vi "Set Adv Mov wrapper.vi"(8 "error in (no error)":errorcluster caption="错误输入（无错误）", 9 "pAdvMovObj":T1, 10 "dwCanNodeId":u32, 11 "dwDevIndex":u32) -> (0 "error out":errorcluster caption="错误输出", 1 "pAdvMovObj out":T1, 3 "function return":u32)   [LabVIEW 2016, in "UISimCanFunc_wrapper.lvlib"]
doc: "_declspec (dllexport) DWORD SetAdvMov_wrapper(DWORD dwDevIndex, DWORD dwCanNodeId, P_ADV_MOVE_PARA_OBJ pAdvMovObj);"
uses:
  <userlib>/UISimCanFunc_wrapper/UISimCanFunc_wrapper.lvlib
  <userlib>/UISimCanFunc_wrapper/UISimCanFunc_wrapper.dll
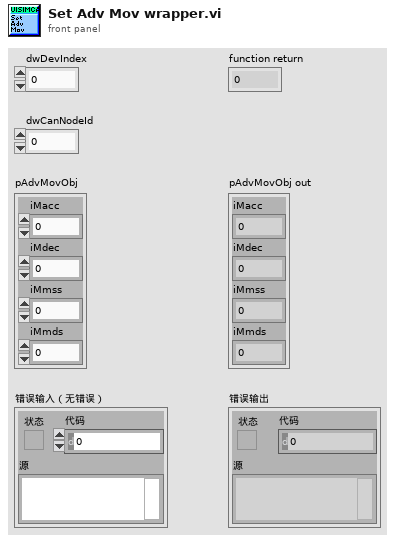
[diagram p1: front panel]
types:
  T1 = cluster{"iMacc":i32, "iMdec":i32, "iMmss":i32, "iMmds":i32}
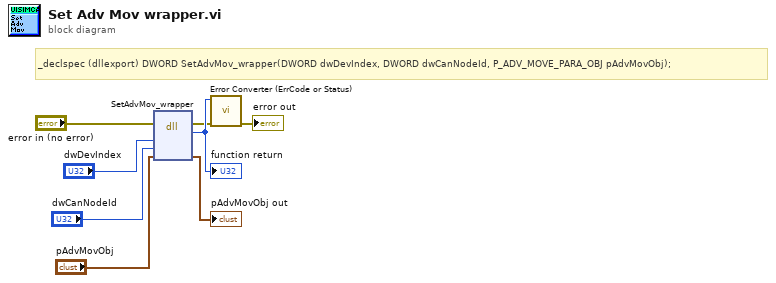
[diagram p0: block diagram]
diagram:
  # "_declspec (dllexport) DWORD SetAdvMov_wrapper(DWORD dwDevIndex, DWORD dwCanNodeId, P_ADV_MOVE_PARA_OBJ pAdvMovObj);"
  n1 = dll-call lib="C:/Program Files (x86)/National Instruments/LabVIEW 2016/user.lib/UISimCanFunc_wrapper/UISimCanFunc_wrapper.*" fn="SetAdvMov_wrapper"(error in="error in (no error)", "dwDevIndex"="dwDevIndex", "dwCanNodeId"="dwCanNodeId", "pAdvMovObj"="pAdvMovObj") -> (error out=w2:errorcluster, w8:u32, "pAdvMovObj"=→"pAdvMovObj out":T1)  [unwired: 4 in, 1 out]
  "function return" <- w8
  n2 = call <userlib>:"Error Converter (ErrCode or Status).vi"("error in (no error)"=w2, "error code"=w8) -> ("error out"=→"error out":errorcluster)  [unwired: 9 in]
